vi "Configure Channel (AIDI Normal).vi"(0 "VISA resource name":refnum<visa-resource-name>, 5 "Channel (0001)":string="0001", 7 "Enable Channel (True)":bool=TRUE, 9 "Span":T1={"DI Type (0 : LVL)"=0, "Lower Span (0)"=0, "Upper Span (1)"=1} {"Upper Span (1)" min=-99999 max=99999 step=1; "Lower Span (0)" min=-99999 max=99999 step=1; "DI Type (0 : LVL)" items=["LVL", "DI"]}, 11 "error in (no error)":errorcluster) -> (4 "VISA resource name out":refnum<visa-resource-name>, 6 "Channel":string, 15 "error out":errorcluster)   [LabVIEW 2020, in "Yokogawa GX Series.lvlib"]
doc: "Sets the input range as Contact.\n\nCommand: SRangeAI"
uses:
  <instrlib>/Yokogawa GX Series/Yokogawa GX Series.lvlib
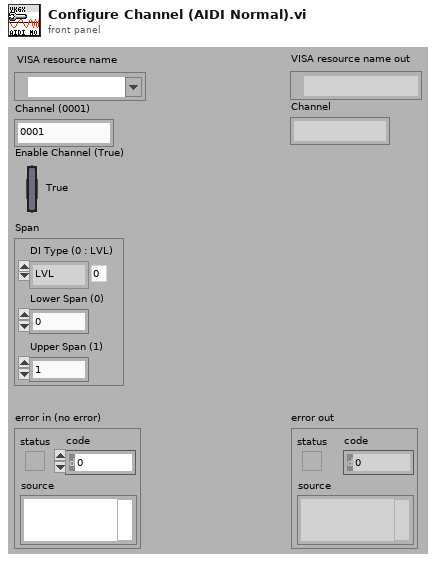
[diagram p1: front panel]
types:
  T1 = cluster{"DI Type (0 : LVL)":i32, "Lower Span (0)":i32, "Upper Span (1)":i32}
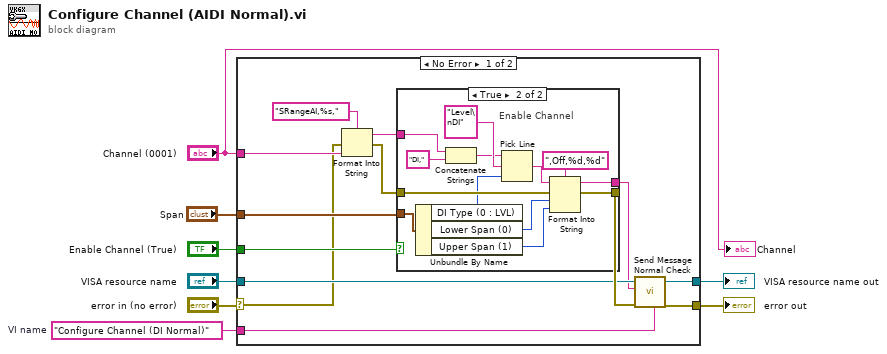
[diagram p0: block diagram]
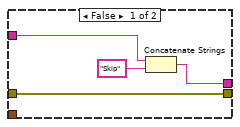
[diagram p2: hidden frame]
diagram:
  w4 = "Configure Channel (DI Normal)"  # VI name
  n1 = case shown="No Error" "error in (no error)" {
    selector: "error in (no error)" -> [w9 w39]
    tunnel: "Enable Channel (True)" -> [w18 _]
    tunnel: [w17 w40] -> w7
    tunnel: [w16 w39] -> w6
    tunnel: "VISA resource name" -> [w14 w40]
    tunnel: w4 -> [w12 _]
    tunnel: "Span" -> [w11 _]
    tunnel: "Channel (0001)" -> [w10 _]
    frame No Error {
      n2 = Format Into String(format string="SRangeAI,%s,", error in=w9, w10) -> (resulting string=w19:string, error out=w20:errorcluster)  [unwired: 1 in]
      n3 = case shown="True" w18 {
        tunnel: w20 -> [w22 w37]
        tunnel: [w22 w35] -> w15
        tunnel: w19 -> [w23 w33]
        tunnel: [w24 w30] -> w13
        tunnel: w11 -> [_ w29]
        frame False {
          n4 = Concatenate Strings(w23, "Skip") -> (w24:string)
        }
        frame True {
          # "Enable Channel"
          n5 = Unbundle By Name(w29) -> ("DI Type (0 : LVL)"=w28:i32, "Lower Span (0)"=w27:i32, "Upper Span (1)"=w26:i32)
          n6 = Concatenate Strings(w33, "DI,") -> (w31:string)
          n7 = Pick Line(string ("")=w31, multi-line string="Level\nDI", line index=w28) -> (output string=w34:string)
          n8 = Format Into String(format string=",Off,%d,%d", initial string=w34, error in=w37, w27, w26) -> (resulting string=w30:string, error out=w35:errorcluster)
        }
      }
      n9 = call <instrlib>:"Send Message Normal Check.vi"("Source (\"\")"=w12, "error in (no error)"=w15, "Send Message (\"\")"=w13, "VISA resource name"=w14) -> ("error out"=w16:errorcluster, "VISA resource name out"=w17:refnum<visa-resource-name>)  [unwired: 2 in, 4 out]
    }
    frame Error {
    }
  }
  "error out" <- w6
  "VISA resource name out" <- w7
  "Channel" <- "Channel (0001)"
